vi "SetNetworkAdaptersSettings.vi"(8 "error in (no error)":errorcluster, 10 "NetworkSettings":T1[](array[typedef]) {"IP Address Request Mode" items=["Static"=1, "DHCP/Link Local"=2, "Link-Local Only"=4, "DHCP Only"=8]; "Adapter Mode" items=["Disabled"=1, "TCP/IP Ethernet"=2, "Deterministic"=4, "EtherCAT"=8, "TCP/IP WLAN Connect"=32, "TCP/IP WLAN Create"=64]}, 11 "Qbus in":refnum<class "Qbus.lvclass">) -> (0 "error out":errorcluster)   [LabVIEW 2017, in "USBDrive.lvlib"]
uses:
  <vilib>/addons/InsightCM/Devices/Shared/Common/USBDrive/USBDrive.lvlib
  <vilib>/addons/SystemInfoProcess/controls/NetworkAdapterSettings.ctl
  <vilib>/addons/Qbus/Qbus.lvclass
  <vilib>/addons/PointValueMap/subVIs/Point_Write_variant.vi
  <vilib>/addons/SystemInfoProcess/SystemInfoProcess.lvlib
  <vilib>/addons/PointValueMap/PointValueMap.lvlib
  <vilib>/addons/InsightCM/Devices/Shared/Common/Controller/Controller.lvlib
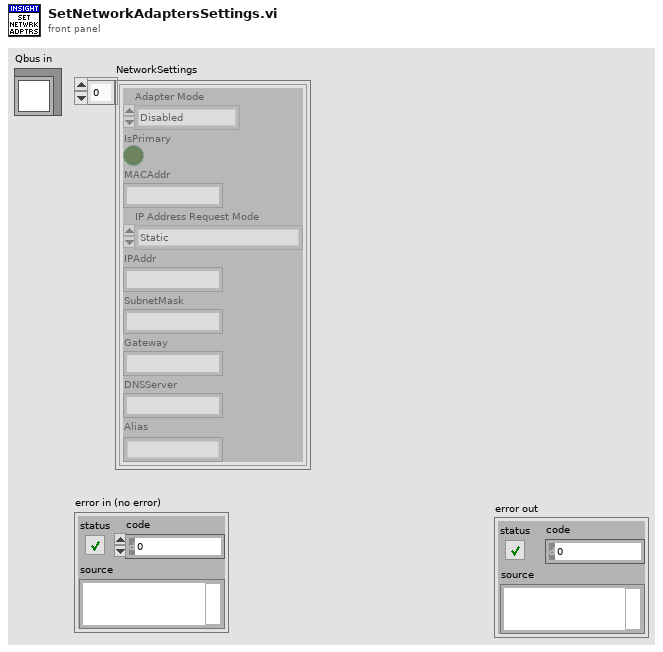
[diagram p1: front panel]
types:
  T1 = typedef "SystemInfoProcess.lvlib/NetworkAdapterSettings.ctl" = cluster{"Adapter Mode":u32, "IsPrimary":bool, "MACAddr":string, "IP Address Request Mode":u32, "IPAddr":string, "SubnetMask":string, "Gateway":string, "DNSServer":string, "Alias":string}
  T2 = typedef "PointValueMap.lvlib/PointMap.ctl" = refnum<data-value>
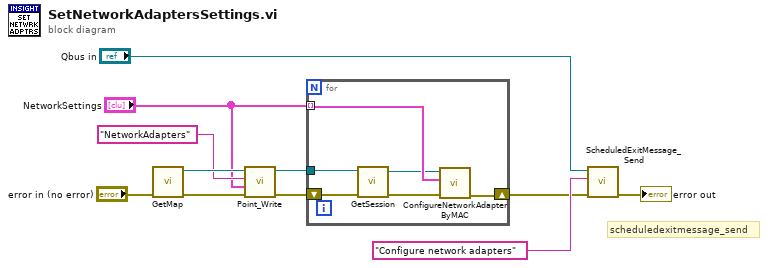
[diagram p0: block diagram]
diagram:
  # "scheduledexitmessage_send"
  n1 = call <vilib>:"GetMap.vi"("error in (no error)"="error in (no error)") -> ("error out"=w9:errorcluster, "SystemInfoMap"=w11:T2)  [unwired: 9 in]
  n2 = call-poly <vilib>:"Point_Write.vi"("Error In"=w9, "Value"="NetworkSettings", "Tag"="NetworkAdapters", "Map"=w11) -> ("Error Out"=w7:errorcluster, "Map Out"=w5:T2)  [unwired: 6 in]
  n3 = for {
    shift-right: [w17] -> w2
    shift-left: w7 -> [w15]
    tunnel: "NetworkSettings" -> [w16] mode=indexing
    tunnel: w5 -> [w12]
    n4 = call <vilib>:"GetSession.vi"("error in (no error)"=w15, "map"=w12) -> ("error out"=w14:errorcluster, "session"=w13:refnum<k21>)  [unwired: 8 in]
    n5 = call <vilib>:"ConfigureNetworkAdapterByMAC.vi"("error in (no error)"=w14, "Network Adapter Settings"=w16, "Session in"=w13) -> ("error out"=w17:errorcluster)  [unwired: 6 in, 2 out]
  }
  n6 = call <vilib>:"ScheduledExitMessage_Send.vi"("error in (no error)"=w2, "scheduled exit reason"="Configure network adapters" ("Tag"), "Qbus in"="Qbus in") -> ("error out"=→"error out":errorcluster)  [unwired: 7 in, 1 out]
